vi "SaveToDrive.vi"(8 "error in":errorcluster, 10 "DataLogger IN":refnum<class "DataLogger.lvclass">, 11 "Cluster IN":T1) -> (0 "error out":errorcluster, 3 "Cluster OUT":T1)   [LabVIEW 2019, in "DataLogger.lvclass"]
doc: "Save to Drive"
uses:
  DataLogger.lvclass
  <vilib>/Utility/file.llb/Write Delimited Spreadsheet (string).vi
  <vilib>/vision/Image Controls.llb/IMAQ Image.ctl
  Common/Controls/AllPartInfo.ctl
  Controls/LocalData_DL.ctl
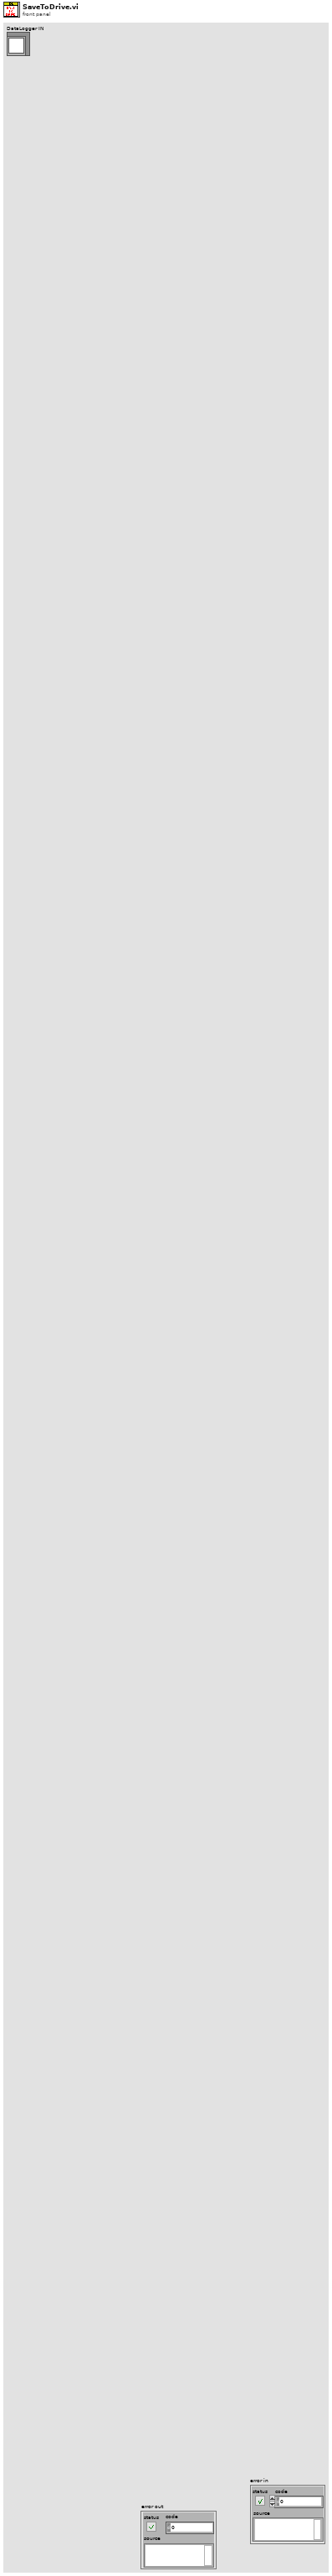
[diagram p1: front panel]
types:
  T1 = typedef "DataLogger.lvclass/LocalData_DL.ctl" = cluster{"Core":cluster{"Current VI Reference":refnum<vi>, "Close Panel on Exit?":bool}, "System Info":cluster{"System Name":string, "System ID":string, "Version":string, "Year":string, "Customer Details":cluster{"Customer Name":string, "Customer ID":string, "Location":string, "No of Shifts":u8, "Shift Details Array":cluster{"Name":string, "Timing":string}[]}, "Software Features":cluster{"IoT Enable":bool, "Datalogging Features":cluster{"Event Data":bool, "Measurement Data":bool, "Statistical Data":bool, "Reel Data":bool, "Failed Measurement Data":bool, "Failed Images":bool}, "IoT":cluster{"SMS Alert Enable":bool, "Email Alert Enable":bool}, "Popup Enable?":cluster{"Fail":bool, "Pause":bool, "Stop":bool}}}, "Part Info":cluster{"Part Name":string, "Rack ID":u8, "Initialize":bool, "StampingMc No":u64, "Operator Name":string, "ReelCount":u64, "TotalCount":u64, "Measurement Names Array":string[], "Measurement ID Array":u16[], "Spec Values Array":cluster{"LCL":dbl, "UCL":dbl, "LSL":dbl, "USL":dbl, "Nominal Value":dbl}[], "Camera Name Array":string[], "Measurement Enable/Disable Array":bool[], "Number of Measurements":i32}, "Fail Counter(For Event Details)":i32, "Event Details":cluster{"Event Name":string, "Event Time":string, "Event Reason":string, "Previous Event Name":string, "Previous Event Time":string}, "StatisticalInfo":string[][], "BatchInfo":cluster{"BatchPassCount":u64, "BatchFailCount":u64}, "Failure Details":cluster{"Fail Time Stamp":u64, "ControlPFArray":bool[], "SpecificationPFArray":dbl[], "Rack ID":u8, "Failed Image Array":T2[], "Fail Date":string, "Fail Time":string, "Fail Reason":string}, "SaveFailedImageCounter":i32, "AllPartInfoArray":T3, "Status":bool, "SpecValues(ForUpdate)":cluster{"LCL":dbl, "UCL":dbl, "LSL":dbl, "USL":dbl, "Nominal Value":dbl}, "AddSuccessfull":bool, "CurrentStateMessage":string, "IoTDetailsCounter":bool, "InitialUpdate":bool, "ResetUpdate":bool, "SetCounter":cluster{"MeasurementDetailsSetCounter":i32, "BatchDetailsSetCounter":i32, "FailureDetailsSetCounter":i32, "EventDetailsSetCounter":i32}, "IndexCounter":cluster{"MeasurementDetailsIndexCounter":i32, "BatchDetailsIndexCounter":i32, "FailureDetailsIndexCounter":i32, "EventDetailsIndexCounter":i32}, "Details2D":cluster{"MeasurementDetails(2D)":string[][], "BatchDetails(2D)":string[][], "FailureDetails(2D)":string[][], "EventDetails(2D)":string[][]}, "IDs":cluster{"Stamping McID":string, "Inspection McID":string, "BatchID":string, "FailID":string}, "Reel Info":cluster{"Reel No":u64, "Reel Start Time Stamp":u64}, "ExcelData":cluster{"StripPath":bool, "ReelCounterPerPart":i32, "FilePaths":cluster{"EventsFilePath":path, "FailFilePath":path, "ReelFilePath":path, "StatisticalFilePath":path}, "ExcelSheetCounterPerReel":cluster{"EventsSheetCounter":u32, "FailSheetCounter":u32, "StatisticalSheetCounter":u32, "ReelSheetCounter":u32}, "CreateNewExcel":cluster{"CreateNewEventsExcel":bool, "CreateNewFailExcel":bool, "CreateNewStatisticalExcel":bool, "CreateNewReelExcel":bool}, "RecordsInExcelCounter":cluster{"EventsRecordsCounter":u32, "FailRecordsCounter":u32, "ReelRecordsCounter":u32, "StatisticalRecordsCounter":u32}}, "SaveAck":cluster{"Loop1":bool, "Loop2":bool}, "Shift Statistical Info":cluster{"Shift Name":string, "Shift Timing":string, "Shift End Date":string, "Statistical Shift Data":cluster{"PartName":string, "MeasurementNames":string[], "Statistical Parameters":string[][]}[]}}
  T2 = typedef "IMAQ Image.ctl" = refnum<image>
  T3 = typedef "AllPartInfo.ctl" = cluster{"PartName":string, "NumberOfRacks":u8, "MeasurementIDsArray":u16[], "MeasurementNamesArray":string[], "SpecValuesArray":cluster{"LCL":dbl, "UCL":dbl, "LSL":dbl, "USL":dbl, "NominalValue":dbl}[]}[]
  T4 = cluster{"Part Name":string, "Reel Number":u64, "Reel start time stamp":u64, "Image array":T2[], "Camera Names":string[], "FailID":string}
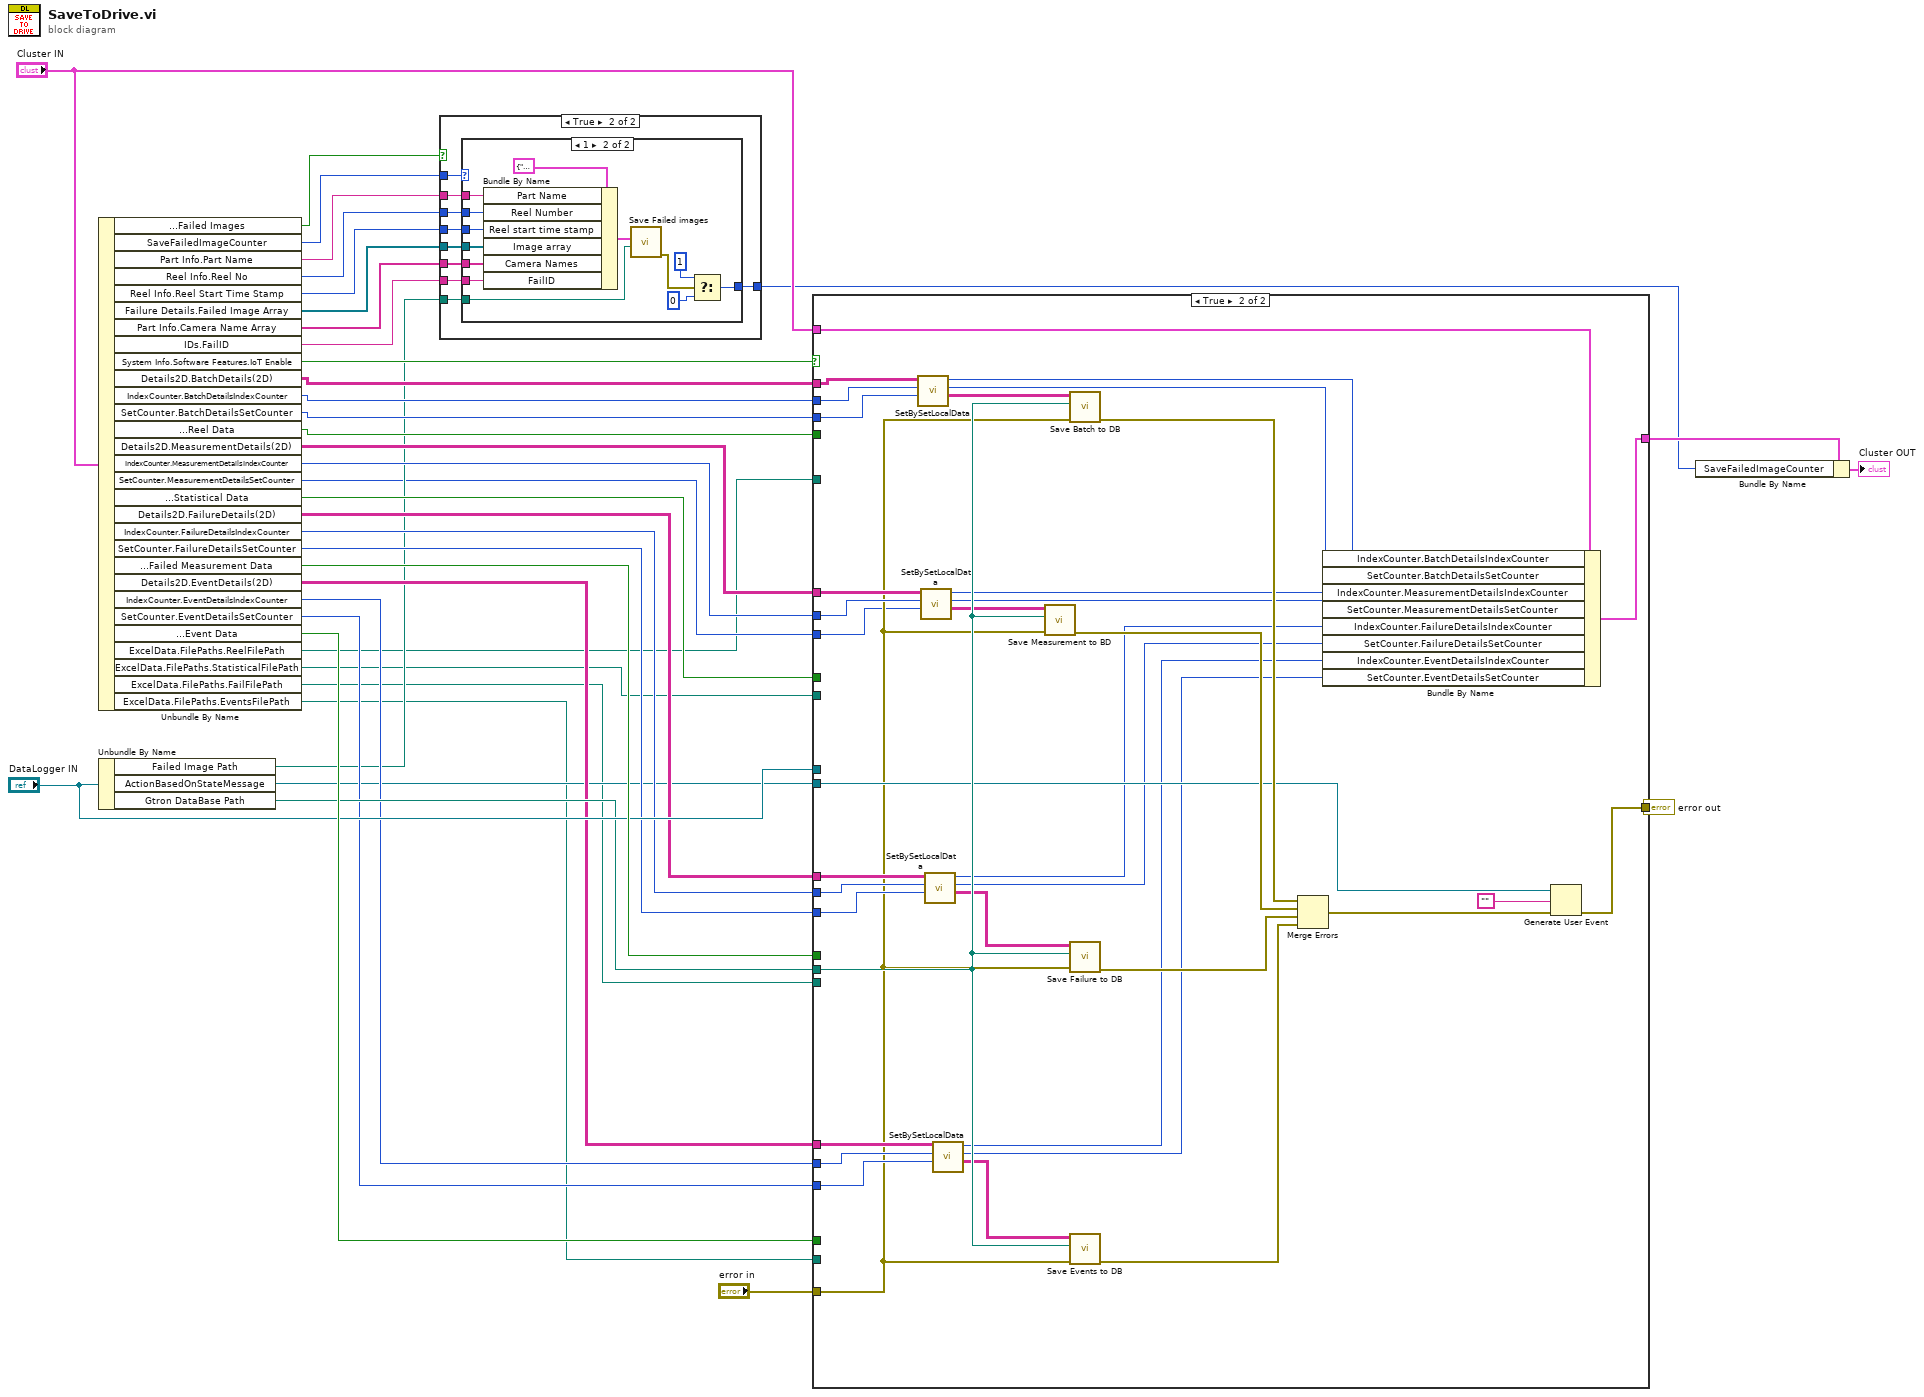
[diagram p0: block diagram]
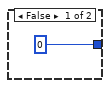
[diagram p2: hidden frame]
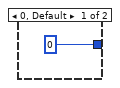
[diagram p3: hidden frame]
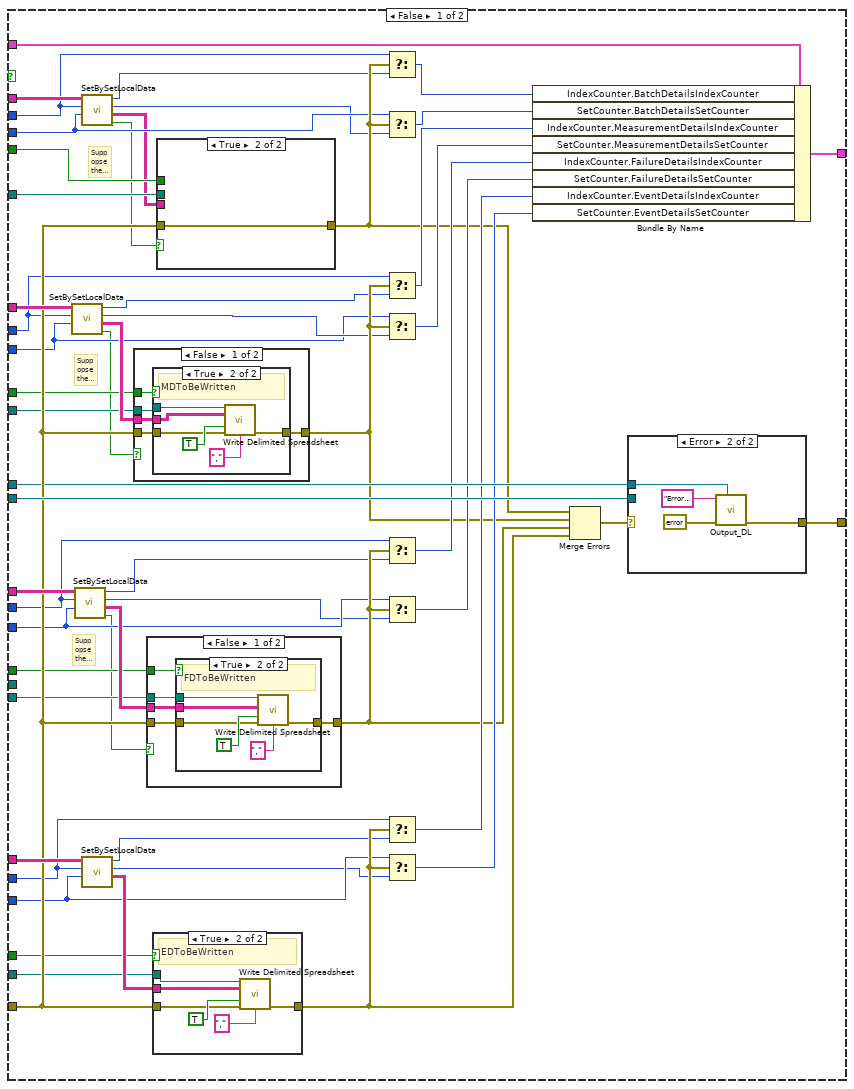
[diagram p4: hidden frame]
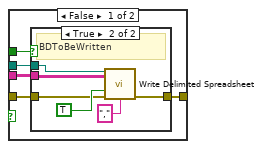
[diagram p6: hidden frame]
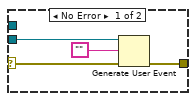
[diagram p12: hidden frame]
diagram:
  n1 = Unbundle By Name("Cluster IN") -> ("System Info.Software Features.Datalogging Features.Failed Images"=w11:bool, "SaveFailedImageCounter"=w10:i32, "Part Info.Part Name"=w17:string, "Reel Info.Reel No"=w16:u64, "Reel Info.Reel Start Time Stamp"=w15:u64, "Failure Details.Failed Image Array"=w14:T2[], "Part Info.Camera Name Array"=w13:string[], "IDs.FailID"=w12:string, "System Info.Software Features.IoT Enable"=w22:bool, "Details2D.BatchDetails(2D)"=w39:string[][], "IndexCounter.BatchDetailsIndexCounter"=w20:i32, "SetCounter.BatchDetailsSetCounter"=w21:i32, "System Info.Software Features.Datalogging Features.Reel Data"=w19:bool, "Details2D.MeasurementDetails(2D)"=w23:string[][], "IndexCounter.MeasurementDetailsIndexCounter"=w24:i32, "SetCounter.MeasurementDetailsSetCounter"=w5:i32, "System Info.Software Features.Datalogging Features.Statistical Data"=w38:bool, "Details2D.FailureDetails(2D)"=w25:string[][], "IndexCounter.FailureDetailsIndexCounter"=w26:i32, "SetCounter.FailureDetailsSetCounter"=w27:i32, "System Info.Software Features.Datalogging Features.Failed Measurement Data"=w35:bool, "Details2D.EventDetails(2D)"=w28:string[][], "IndexCounter.EventDetailsIndexCounter"=w29:i32, "SetCounter.EventDetailsSetCounter"=w30:i32, "System Info.Software Features.Datalogging Features.Event Data"=w36:bool, "ExcelData.FilePaths.ReelFilePath"=w4:path, "ExcelData.FilePaths.StatisticalFilePath"=w3:path, "ExcelData.FilePaths.FailFilePath"=w2:path, "ExcelData.FilePaths.EventsFilePath"=w1:path)
  n2 = Unbundle By Name("DataLogger IN") -> ("Failed Image Path"=w6:path, "ActionBasedOnStateMessage"=w18:refnum<user-event>, "Gtron DataBase Path"=w31:path)
  n3 = case shown="True" w11 {
    tunnel: w17 -> [_ w49]
    tunnel: w16 -> [_ w48]
    tunnel: w15 -> [_ w47]
    tunnel: w14 -> [_ w46]
    tunnel: w13 -> [_ w45]
    tunnel: w12 -> [_ w44]
    tunnel: w10 -> [_ w43]
    tunnel: [0 w42] -> w8
    tunnel: w6 -> [_ w41]
    frame False {
    }
    frame True {
      n4 = case shown="1" w43 {
        tunnel: w49 -> [_ w62]
        tunnel: w48 -> [_ w61]
        tunnel: w47 -> [_ w60]
        tunnel: w46 -> [_ w59]
        tunnel: w45 -> [_ w58]
        tunnel: w44 -> [_ w57]
        tunnel: [0 w55] -> w42
        tunnel: w41 -> [_ w52]
        frame 0, Default {
        }
        frame 1 {
          n5 = Bundle By Name(cluster=T4 {"Part Name"="", "Reel Number"=0, "Reel start time stamp"=0, "Image array"=[], "Camera Names"=[], "FailID"=""} ("Image Info"), "Part Name"=w62, "Reel Number"=w61, "Reel start time stamp"=w60, "Image array"=w59, "Camera Names"=w58, "FailID"=w57) -> (w63:T4)
          n6 = call "Save Failed images.vi"("Failed Image path"=w52, "Image Info"=w63) -> ("error out"=w56:errorcluster)  [unwired: 9 in]
          n7 = Select(t=1, s=w56, f=0) -> (s? t:f=w55:i32)
        }
      }
    }
  }
  n8 = case shown="True" w22 {
    tunnel: w20 -> [w83 w207]
    tunnel: w21 -> [w81 w206]
    tunnel: w39 -> [w115 w205]
    tunnel: w23 -> [w114 w190]
    tunnel: w24 -> [w79 w189]
    tunnel: w5 -> [w76 w172]
    tunnel: w25 -> [w113 w188]
    tunnel: w26 -> [w75 w187]
    tunnel: w27 -> [w73 w186]
    tunnel: w28 -> [w112 w185]
    tunnel: w29 -> [w71 w184]
    tunnel: w30 -> [w69 w183]
    tunnel: w31 -> [_ w201]
    tunnel: [w116 w200] -> w9
    tunnel: "Cluster IN" -> [w117 w199]
    tunnel: "error in" -> [w105 w173]
    tunnel: [w106 w198] -> w33
    tunnel: w18 -> [w107 w192]
    tunnel: w1 -> [w104 _]
    tunnel: w2 -> [w103 _]
    tunnel: w4 -> [w102 _]
    tunnel: w3 -> [w101 _]
    tunnel: "DataLogger IN" -> [w96 _]
    tunnel: w19 -> [w100 _]
    tunnel: w38 -> [w99 _]
    tunnel: w35 -> [w98 _]
    tunnel: w36 -> [w97 _]
    frame False {
      # "Suppopse the user presses softawareExit before inspection starts.So by that time fail,reel and statistical file path wont be there.So when save comes\nduring SoftwareExit,DL will try to write fail,reel and statistical data but there is still no file path for saving.This will create an error."
      # "Suppopse the user presses softawareExit before inspection starts.So by that time fail,reel and statistical file path wont be there.So when save comes\nduring SoftwareExit,DL will try to write fail,reel and statistical data but there is still no file path for saving.This will create an error."
      # "Suppopse the user presses softawareExit before inspection starts.So by that time fail,reel and statistical file path wont be there.So when save comes\nduring SoftwareExit,DL will try to write fail,reel and statistical data but there is still no file path for saving.This will create an error."
      n9 = call "SetBySetLocalData.vi"("SetCounterIN"=w76, "IndexCounterIN"=w79, "DataIN"=w114) -> ("Empty DataOUT"=w65:bool, "DataOUT"=w111:string[][], "SetCounterOUT"=w77:i32, "IndexCounterOUT"=w78:i32)  [unwired: 5 in]
      n10 = call "SetBySetLocalData.vi"("SetCounterIN"=w73, "IndexCounterIN"=w75, "DataIN"=w113) -> ("Empty DataOUT"=w64:bool, "DataOUT"=w110:string[][], "SetCounterOUT"=w72:i32, "IndexCounterOUT"=w74:i32)  [unwired: 5 in]
      n11 = call "SetBySetLocalData.vi"("SetCounterIN"=w81, "IndexCounterIN"=w83, "DataIN"=w115) -> ("Empty DataOUT"=w66:bool, "DataOUT"=w67:string[][], "SetCounterOUT"=w80:i32, "IndexCounterOUT"=w82:i32)  [unwired: 5 in]
      n12 = call "SetBySetLocalData.vi"("SetCounterIN"=w69, "IndexCounterIN"=w71, "DataIN"=w112) -> ("DataOUT"=w109:string[][], "SetCounterOUT"=w68:i32, "IndexCounterOUT"=w70:i32)  [unwired: 5 in, 1 out]
      n13 = case shown="False" w65 {
        tunnel: w111 -> [w142 _]
        tunnel: w105 -> [w141 w150]
        tunnel: w101 -> [w140 _]
        tunnel: w99 -> [w139 _]
        tunnel: [w138 w150] -> w86
        frame False {
          n14 = case shown="True" w139 {
            tunnel: [w143 w149] -> w138
            tunnel: w142 -> [_ w147]
            tunnel: w141 -> [w143 w145]
            tunnel: w140 -> [_ w144]
            frame False {
              # "MDNotToBeWritten"
            }
            frame True {
              # "MDToBeWritten"
              n15 = call-poly <vilib>:"Write Delimited Spreadsheet.vi"("file path (dialog if empty)"=w144, "2D data"=w147, "append to file? (new file:F)"=TRUE ("append to file? (F)"), "error in (no error)"=w145, "delimiter (\\t)"="," ("delimiter (\\t)")) -> ("error out"=w149:errorcluster)  [unwired: 9 in, 1 out]
            }
          }
        }
        frame True {
        }
      }
      n16 = case shown="False" w64 {
        tunnel: w110 -> [w155 _]
        tunnel: w105 -> [w154 w163]
        tunnel: w103 -> [w153 _]
        tunnel: w98 -> [w152 _]
        tunnel: [w151 w163] -> w85
        frame False {
          n17 = case shown="True" w152 {
            tunnel: [w156 w161] -> w151
            tunnel: w155 -> [_ w160]
            tunnel: w154 -> [w156 w158]
            tunnel: w153 -> [_ w157]
            frame False {
              # "FDNotToBeWritten"
            }
            frame True {
              # "FDToBeWritten"
              n18 = call-poly <vilib>:"Write Delimited Spreadsheet.vi"("file path (dialog if empty)"=w157, "2D data"=w160, "append to file? (new file:F)"=TRUE ("append to file? (F)"), "error in (no error)"=w158, "delimiter (\\t)"="," ("delimiter (\\t)")) -> ("error out"=w161:errorcluster)  [unwired: 9 in, 1 out]
            }
          }
        }
        frame True {
        }
      }
      n19 = case shown="True" w97 {
        tunnel: [w118 w124] -> w84
        tunnel: w109 -> [_ w122]
        tunnel: w105 -> [w118 w120]
        tunnel: w104 -> [_ w119]
        frame False {
          # "EDNotToBeWritten"
        }
        frame True {
          # "EDToBeWritten"
          n20 = call-poly <vilib>:"Write Delimited Spreadsheet.vi"("file path (dialog if empty)"=w119, "2D data"=w122, "append to file? (new file:F)"=TRUE ("append to file? (F)"), "error in (no error)"=w120, "delimiter (\\t)"="," ("delimiter (\\t)")) -> ("error out"=w124:errorcluster)  [unwired: 9 in, 1 out]
        }
      }
      n21 = case shown="True" w66 {
        tunnel: w67 -> [w129 _]
        tunnel: w105 -> [w128 w137]
        tunnel: w102 -> [w127 _]
        tunnel: w100 -> [w126 _]
        tunnel: [w125 w137] -> w87
        frame False {
          n22 = case shown="True" w126 {
            tunnel: [w130 w135] -> w125
            tunnel: w129 -> [_ w134]
            tunnel: w128 -> [w130 w132]
            tunnel: w127 -> [_ w131]
            frame False {
              # "BDNotToBeWritten"
            }
            frame True {
              # "BDToBeWritten"
              n23 = call-poly <vilib>:"Write Delimited Spreadsheet.vi"("file path (dialog if empty)"=w131, "2D data"=w134, "append to file? (new file:F)"=TRUE ("append to file? (F)"), "error in (no error)"=w132, "delimiter (\\t)"="," ("delimiter (\\t)")) -> ("error out"=w135:errorcluster)  [unwired: 9 in, 1 out]
            }
          }
        }
        frame True {
        }
      }
      n24 = Select(t=w83, s=w87, f=w82) -> (s? t:f=w95:i32)
      n25 = Select(t=w81, s=w87, f=w80) -> (s? t:f=w94:i32)
      n26 = Select(t=w79, s=w86, f=w78) -> (s? t:f=w93:i32)
      n27 = Select(t=w76, s=w86, f=w77) -> (s? t:f=w92:i32)
      n28 = Select(t=w75, s=w85, f=w74) -> (s? t:f=w91:i32)
      n29 = Select(t=w73, s=w85, f=w72) -> (s? t:f=w90:i32)
      n30 = Select(t=w71, s=w84, f=w70) -> (s? t:f=w89:i32)
      n31 = Select(t=w69, s=w84, f=w68) -> (s? t:f=w88:i32)
      n32 = Bundle By Name(cluster=w117, "IndexCounter.BatchDetailsIndexCounter"=w95, "SetCounter.BatchDetailsSetCounter"=w94, "IndexCounter.MeasurementDetailsIndexCounter"=w93, "SetCounter.MeasurementDetailsSetCounter"=w92, "IndexCounter.FailureDetailsIndexCounter"=w91, "SetCounter.FailureDetailsSetCounter"=w90, "IndexCounter.EventDetailsIndexCounter"=w89, "SetCounter.EventDetailsSetCounter"=w88) -> (w116:T1)
      n33 = Merge Errors(w87, w86, w85, w84) -> (w108:errorcluster)
      n34 = case shown="Error" w108 {
        selector: w108 -> [w166 _]
        tunnel: w107 -> [w165 _]
        tunnel: [w164 w168] -> w106
        tunnel: w96 -> [_ w171]
        frame No Error {
          n35 = Generate User Event(user event=w165, event data cluster="" ("event data"), error in=w166) -> (error out=w164:errorcluster)  [unwired: 1 in, 1 out]
        }
        frame Error {
          n36 = call "Output_DL.vi"("Private Data"=w171, "error in (no error)"=errorcluster {"status"=FALSE, "code"=0, "source"=""}, "State"="ErrorPopUp") -> ("error out"=w168:errorcluster)  [unwired: 8 in]
        }
      }
    }
    frame True {
      n37 = call "SetBySetLocalData.vi"("SetCounterIN"=w206, "IndexCounterIN"=w207, "DataIN"=w205) -> ("DataOUT"=w202:string[][], "SetCounterOUT"=w204:i32, "IndexCounterOUT"=w203:i32)  [unwired: 5 in, 1 out]
      n38 = call "SetBySetLocalData.vi"("SetCounterIN"=w172, "IndexCounterIN"=w189, "DataIN"=w190) -> ("DataOUT"=w176:string[][], "SetCounterOUT"=w181:i32, "IndexCounterOUT"=w182:i32)  [unwired: 5 in, 1 out]
      n39 = call "SetBySetLocalData.vi"("SetCounterIN"=w186, "IndexCounterIN"=w187, "DataIN"=w188) -> ("DataOUT"=w175:string[][], "SetCounterOUT"=w179:i32, "IndexCounterOUT"=w180:i32)  [unwired: 5 in, 1 out]
      n40 = call "SetBySetLocalData.vi"("SetCounterIN"=w183, "IndexCounterIN"=w184, "DataIN"=w185) -> ("DataOUT"=w174:string[][], "SetCounterOUT"=w177:i32, "IndexCounterOUT"=w178:i32)  [unwired: 5 in, 1 out]
      n41 = call "Save Measurement to BD.vi"("error in"=w173, "GTron DB"=w201, "Values"=w176) -> ("error out"=w196:errorcluster)  [unwired: 8 in]
      n42 = call "Save Batch to DB.vi"("error in"=w173, "GTron DB"=w201, "Values"=w202) -> ("error out"=w197:errorcluster)  [unwired: 8 in]
      n43 = call "Save Failure to DB.vi"("error in"=w173, "GTron DB"=w201, "Array"=w175) -> ("error out"=w195:errorcluster)  [unwired: 8 in]
      n44 = call "Save Events to DB.vi"("Array"=w174, "db file"=w201, "error in"=w173) -> ("error out"=w194:errorcluster)  [unwired: 7 in]
      n45 = Merge Errors(w197, w196, w195, w194) -> (w193:errorcluster)
      n46 = Bundle By Name(cluster=w199, "IndexCounter.BatchDetailsIndexCounter"=w203, "SetCounter.BatchDetailsSetCounter"=w204, "IndexCounter.MeasurementDetailsIndexCounter"=w182, "SetCounter.MeasurementDetailsSetCounter"=w181, "IndexCounter.FailureDetailsIndexCounter"=w180, "SetCounter.FailureDetailsSetCounter"=w179, "IndexCounter.EventDetailsIndexCounter"=w178, "SetCounter.EventDetailsSetCounter"=w177) -> (w200:T1)
      n47 = Generate User Event(user event=w192, event data cluster="" ("event data"), error in=w193) -> (error out=w198:errorcluster)  [unwired: 1 in, 1 out]
    }
  }
  "error out" <- w33
  n48 = Bundle By Name(cluster=w9, "SaveFailedImageCounter"=w8) -> (→"Cluster OUT":T1)
